vi "Connect_EventRefOut_Void.vi"(8 "Error In":errorcluster, 10 "Signal Signature":string, 11 "Sender In":refnum<class "LQObject.lvclass">) -> (0 "Error Out":errorcluster, 2 "Void Signal":refnum<user-event>, 3 "Sender Out":refnum<class "LQObject.lvclass">)   [LabVIEW 2014, in "LQ Core.lvlib" / "LQCoreEngine.lvclass"]
uses:
  LQCoreEngine.lvclass
  LQObject/LQObject.lvclass
  _Private/Signals and Slots/Connection Action.ctl
  _Private/Signals and Slots/Signal Data Type.ctl
  LQIdentity/LQIdentity.lvclass/LQIdentity.ctl
  LQ Core.lvlib
  LQIdentity/LQIdentity.lvclass
panel:
  # "Copyright (c) 2016 Sze Howe Koh\n\nThis Source Code Form is subject to the terms of the Mozilla Public\nLicense, v. 2.0. If a copy of the MPL was not distributed with this\nfile, You can obtain one at http://mozilla.org/MPL/2.0/."
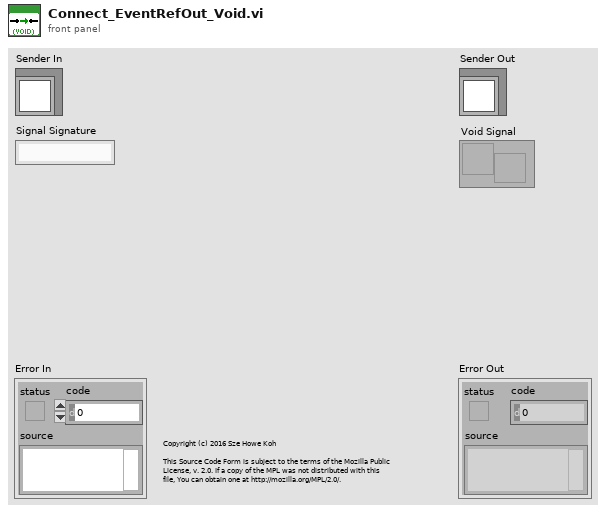
[diagram p1: front panel]
types:
  T1 = typedef "LQ Core.lvlib/LQCoreEngine.lvclass/Signal Data Type.ctl" = enum16{"Void", "Bool", "I32", "DBL", "String"}
  T2 = typedef "LQ Core.lvlib/LQCoreEngine.lvclass/Connection Action.ctl" = enum16{"Init", "Add Connection", "Get Connections", "Clean Up"}
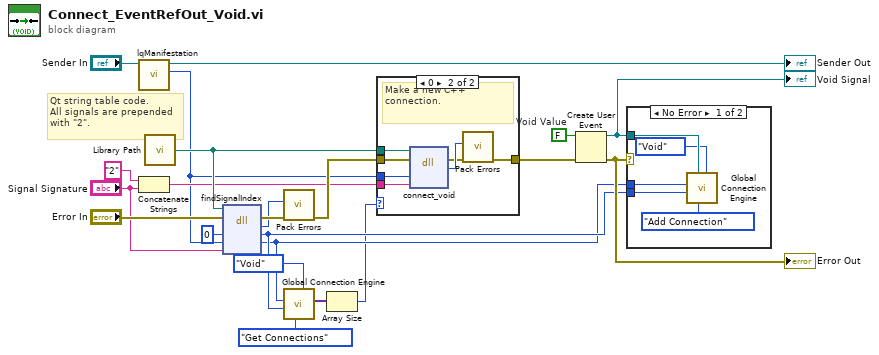
[diagram p0: block diagram]
diagram:
  w5 = FALSE  # Void Value
  # "Qt string table code.\nAll signals are prepended\nwith \"2\"."
  n1 = call "lqManifestation.vi"("LQIdentity in"="Sender In") -> ("Manifestation"=w13:u64, "LQIdentity out"=→"Sender Out":refnum<class "LQObject.lvclass">)  [unwired: 9 in]
  n2 = Concatenate Strings("2" ("string"), "Signal Signature") -> (w15:string)
  n3 = call "Library Path.vi"() -> ("Library Path"=w19:path)
  n4 = dll-call lib="?" fn="findSignalIndex"(path in=w19, error in="Error In", "_retVal"=i64 0 ("retVal"), "_instance"=w13, "normalizedSignal"="Signal Signature") -> (error out=w11:errorcluster, "errorCode"=w10:i32, "_retVal"=w8:i64, "_instance"=w7:u64)  [unwired: 2 in, 1 out]
  n5 = call "Pack Errors.vi"("Error In"=w11, "Error Code"=w10) -> ("Error Out"=w21:errorcluster)  [unwired: 9 in]
  n6 = call "Global Connection Engine.vi"("Receiver Data Type"=Signal_Data_Type."Void", "Connection Action"=Connection_Action."Get Connections", "Signal Index"=w8, "LQObject Manifestation"=w7) -> ("Receiver Channels Out"=w6:variant[])  [unwired: 7 in]
  n7 = Array Size(array=w6) -> (size(s)=w3:i32)
  n8 = case shown="0" w3 {
    tunnel: w15 -> [_ w30]
    tunnel: w19 -> [_ w29]
    tunnel: w13 -> [_ w28]
    tunnel: w21 -> [w23 w27]
    tunnel: [w23 w24] -> w4
    frame Default {
      # "Don't create a duplicate\nconnection."
    }
    frame 0 {
      # "Make a new C++\nconnection."
      n9 = dll-call lib="?" fn="connect_void"(path in=w29, error in=w27, "_instance"=w28, "encodedSignal"=w30) -> (error out=w25:errorcluster, "errorCode"=w26:i32)  [unwired: 3 in, 1 out]
      n10 = call "Pack Errors.vi"("Error In"=w25, "Error Code"=w26) -> ("Error Out"=w24:errorcluster)  [unwired: 9 in]
    }
  }
  n11 = Create User Event(user event datatype=w5, error in=w4) -> (user event=w2:refnum<user-event>, error out=w22:errorcluster)
  "Error Out" <- w22
  "Void Signal" <- w2
  n12 = case shown="No Error" w22 {
    tunnel: w2 -> [w32 _]
    tunnel: w8 -> [w35 _]
    tunnel: w7 -> [w34 _]
    frame No Error {
      n13 = call "Global Connection Engine.vi"("Receiver Data Type"=Signal_Data_Type."Void", "Connection Action"=Connection_Action."Add Connection", "Receiver Channel In"=w32, "Signal Index"=w35, "LQObject Manifestation"=w34) -> ()  [unwired: 6 in, 1 out]
    }
    frame Error {
    }
  }
